vi "Main.vi"() -> ()   [LabVIEW 2015]
uses:
  TypeDefs/Queue Data.ctl
  FGV/Timer Actions.ctl
  SubVIs/App Data.vi
  SubVIs/App Strings.vi
panel:
  in  "Period [s]":dbl
  in  "Device name":tag="myDAQ1"
  out "Time Elapsed":dbl format="%<%M:%S>t"
  out "Status":string
  in  "Time [ms]":dbl
  in  "Frequency":dbl
  in  "Stop Button":bool
  in  "Acquire Button":bool
  out "Waveform Graph":dbl[](graph)
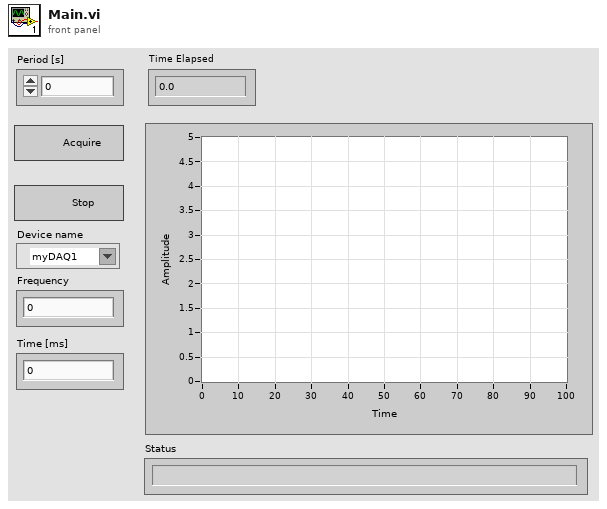
[diagram p1: front panel]
types:
  T1 = typedef "Timer Actions.ctl" = enum16{"Reset", "Get"}
  T2 = typedef "Queue Data.ctl" = cluster{"Action":string}
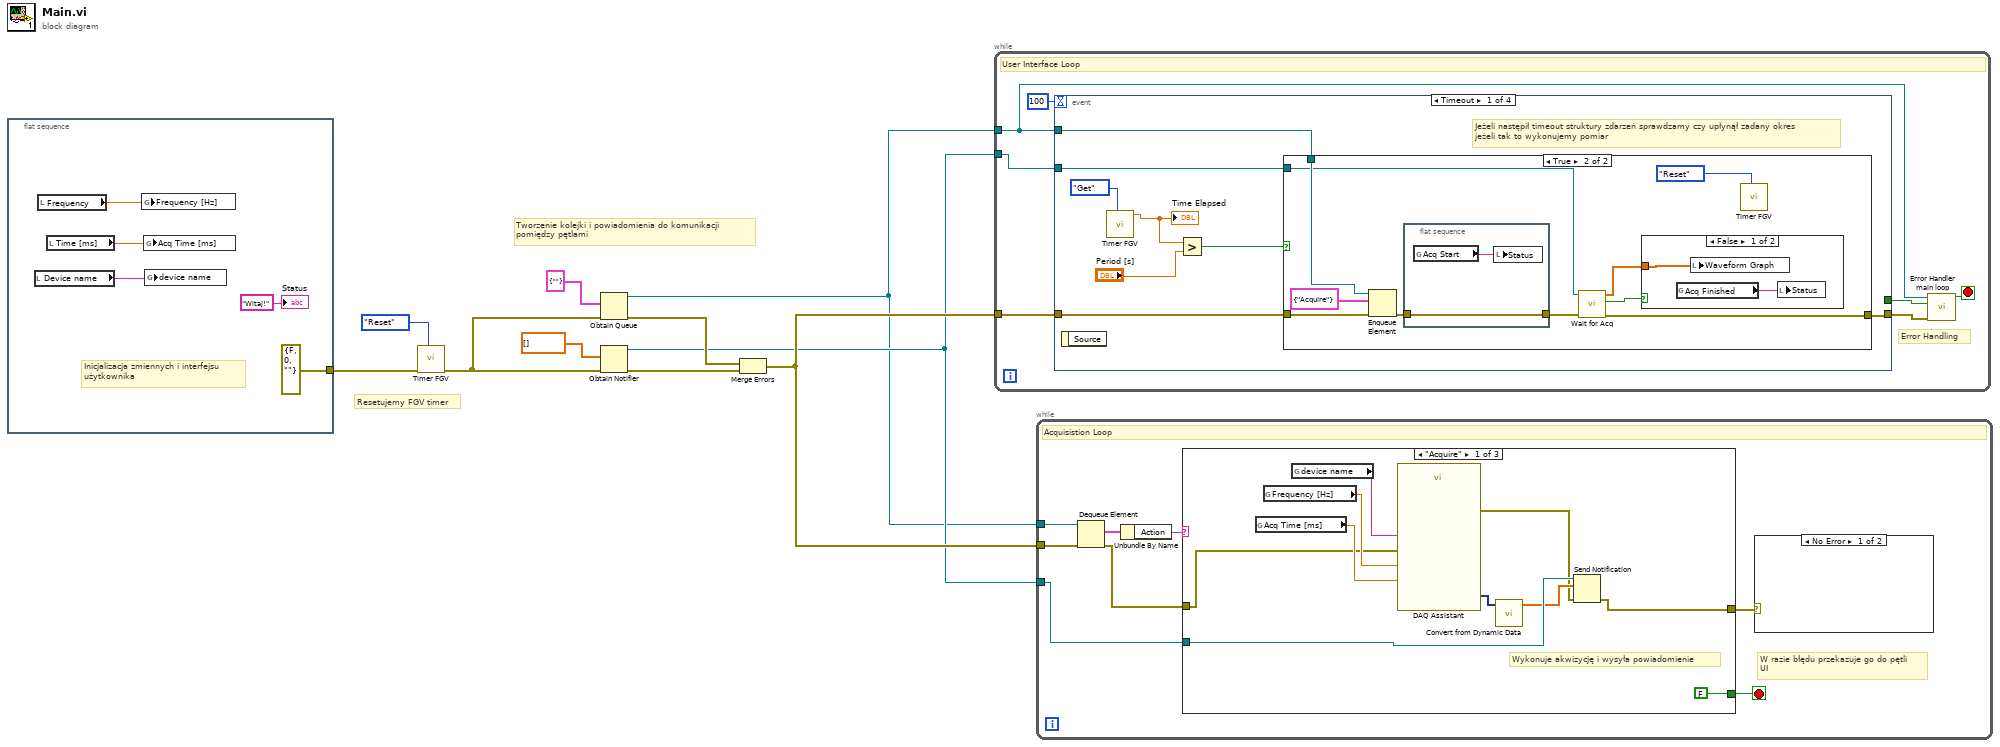
[diagram p0: block diagram]
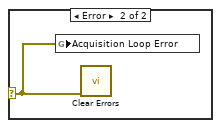
[diagram p2: hidden frame]
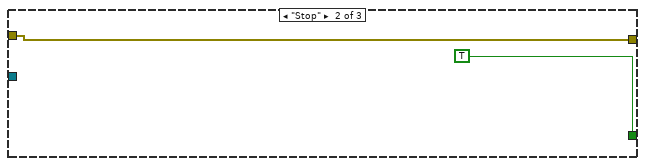
[diagram p3: hidden frame]
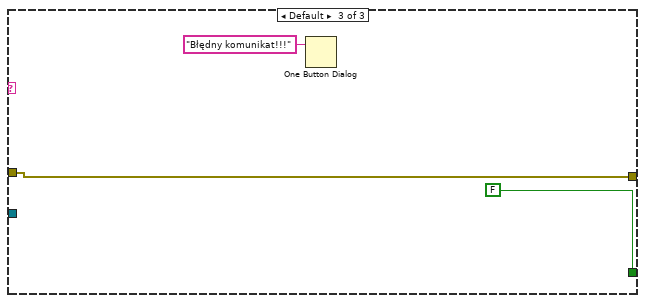
[diagram p4: hidden frame]
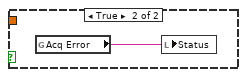
[diagram p6: hidden frame]
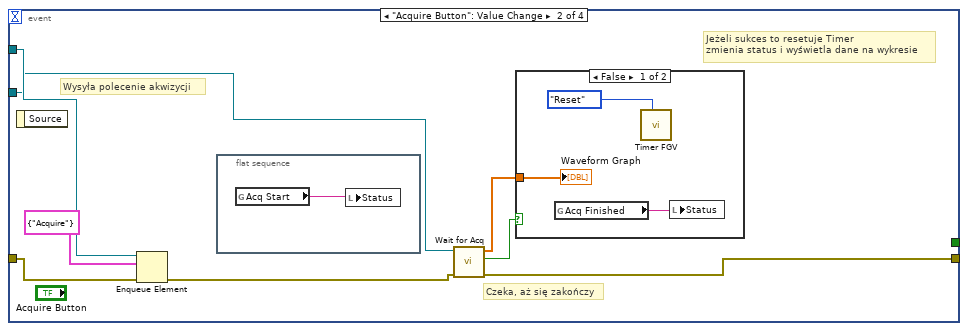
[diagram p7: hidden frame]
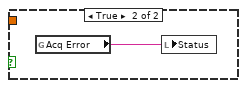
[diagram p8: hidden frame]
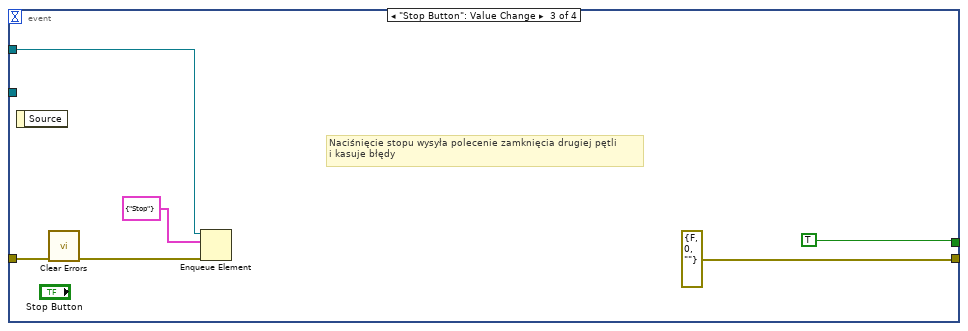
[diagram p9: hidden frame]
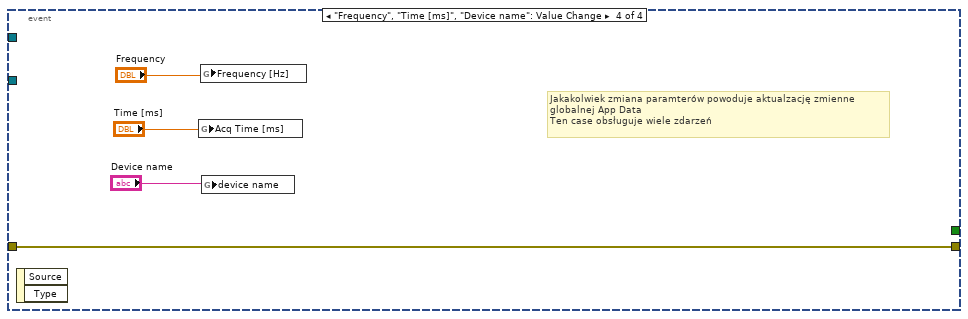
[diagram p10: hidden frame]
diagram:
  # "Resetujemy FGV timer"
  # "Tworzenie kolejki i powiadomienia do komunikacji \npomiędzy pętlami"
  n1 = flat-sequence {
    tunnel: [errorcluster {"status"=FALSE, "code"=0, "source"=""} ("error constant")] -> w3
    frame #0 {
      # "Inicjalizacja zmiennych i interfejsu \nużytkownika"
      n2 = local read "Device name"() -> (w11:tag)
      n3 = local read "Frequency"() -> (w13:dbl)
      n4 = local read "Time [ms]"() -> (w12:dbl)
      n5 = global write "App Data.vi" "Frequency [Hz]"(w13) -> ()
      n6 = global write "App Data.vi" "Acq Time [ms]"(w12) -> ()
      n7 = global write "App Data.vi" "device name"(w11) -> ()
      "Status" <- "Witaj!" ("Status")
    }
  }
  n8 = call "Timer FGV.vi"("Action"=Timer_Actions."Reset", "error in (no error)"=w3) -> ("error out"=w2:errorcluster)  [unwired: 8 in, 1 out]
  n9 = Obtain Queue(element data type=T2 {"Action"=""}, error in (no error)=w2) -> (queue out=w4:refnum<queue>, error out=w9:errorcluster)  [unwired: 3 in, 1 out]
  n10 = Obtain Notifier(notification data type=dbl[] [], error in (no error)=w2) -> (notifier out=w5:refnum<notifier>, error out=w7:errorcluster)  [unwired: 2 in, 1 out]
  n11 = Merge Errors(w9, w7) -> (w6:errorcluster)
  n12 = while {
    tunnel: w6 -> [w21]
    tunnel: w4 -> [w17]
    tunnel: w5 -> [w16]
    stop <- w18 stop-if-true
    # "Error Handling"
    # "User Interface Loop"
    n13 = event shown="[0] Timeout" {
      selector: _ -> [_ _ _ _]
      dyn-events: _ -> [_ _ _ _]
      timeout: 100 -> [_ _ _ _]
      tunnel: w21 -> [w28 w53 w62 w69]
      tunnel: [w27 w48 errorcluster {"status"=FALSE, "code"=0, "source"=""} ("error constant") w69] -> w19
      tunnel: [_ _ TRUE _] -> w20
      tunnel: w17 -> [w24 w54 w60 _]
      tunnel: w16 -> [w23 w50 _ _]
      event Timeout {
        # "Jeżeli następił timeout struktury zdarzeń sprawdzamy czy upłynął zadany okres \njeżeli tak to wykonujemy pomiar"
        n14 = event-data() -> ()  [unwired: 1 in, 1 out]
        n15 = call "Timer FGV.vi"("Action"=Timer_Actions."Get") -> ("Elapsed Time"=w26:dbl)  [unwired: 9 in, 1 out]
        "Time Elapsed" <- w26
        n16 = Greater?(x=w26, y="Period [s]") -> (0:w29:bool)
        n17 = case shown="True" w29 {
          tunnel: w28 -> [w31 w41]
          tunnel: [w31 w34] -> w27
          tunnel: w24 -> [_ w33]
          tunnel: w23 -> [_ w32]
          frame False {
          }
          frame True {
            n18 = Enqueue Element(queue=w33, element=T2 {"Action"="Acquire"}, error in (no error)=w41) -> (error out=w39:errorcluster)  [unwired: 1 in, 2 out]
            n19 = flat-sequence {
              tunnel: w39 -> [w45]
              tunnel: [w45] -> w38
              frame #0 {
                n20 = global read "App Strings.vi" "Acq Start"() -> (w46:string)
                n21 = local write "Status"(w46) -> ()
              }
            }
            n22 = call "Wait for Acq.vi"("error in (no error)"=w38, "Notifier in"=w32) -> ("error out"=w34:errorcluster, "timed out?"=w35:bool, "Array"=w37:dbl[])  [unwired: 7 in]
            n23 = case shown="False" w35 {
              tunnel: w37 -> [w42 _]
              frame False {
                n24 = global read "App Strings.vi" "Acq Finished"() -> (w43:string)
                n25 = local write "Waveform Graph"(w42) -> ()
                n26 = local write "Status"(w43) -> ()
              }
              frame True {
                n27 = global read "App Strings.vi" "Acq Error"() -> (w44:string)
                n28 = local write "Status"(w44) -> ()
              }
            }
            n29 = call "Timer FGV.vi"("Action"=Timer_Actions."Reset") -> ()  [unwired: 9 in, 2 out]
          }
        }
      }
      event "Acquire Button": Value Change {
        # "Jeżeli sukces to resetuje Timer\nzmienia status i wyświetla dane na wykresie"
        # "Czeka, aż się zakończy"
        # "Wysyła polecenie akwizycji"
        n30 = event-data() -> ()  [unwired: 1 in, 1 out]
        n31 = Enqueue Element(queue=w54, element=T2 {"Action"="Acquire"}, error in (no error)=w53) -> (error out=w49:errorcluster)  [unwired: 1 in, 2 out]
        n32 = flat-sequence {
          frame #0 {
            n33 = global read "App Strings.vi" "Acq Start"() -> (w55:string)
            n34 = local write "Status"(w55) -> ()
          }
        }
        n35 = call "Wait for Acq.vi"("error in (no error)"=w49, "Notifier in"=w50) -> ("error out"=w48:errorcluster, "timed out?"=w47:bool, "Array"=w51:dbl[])  [unwired: 7 in]
        n36 = case shown="False" w47 {
          tunnel: w51 -> [w56 _]
          frame False {
            n37 = global read "App Strings.vi" "Acq Finished"() -> (w58:string)
            n38 = call "Timer FGV.vi"("Action"=Timer_Actions."Reset") -> ()  [unwired: 9 in, 2 out]
            n39 = local write "Status"(w58) -> ()
            "Waveform Graph" <- w56
          }
          frame True {
            n40 = global read "App Strings.vi" "Acq Error"() -> (w59:string)
            n41 = local write "Status"(w59) -> ()
          }
        }
      }
      event "Stop Button": Value Change {
        # "Naciśnięcie stopu wysyła polecenie zamknięcia drugiej pętli\ni kasuje błędy"
        n42 = event-data() -> ()  [unwired: 1 in, 1 out]
        n43 = call <vilib>:"Clear Errors.vi"("error in (no error)"=w62) -> ("error out"=w61:errorcluster)  [unwired: 5 in, 1 out]
        n44 = Enqueue Element(queue=w60, element=T2 {"Action"="Stop"}, error in (no error)=w61) -> ()  [unwired: 1 in, 3 out]
      }
      event "Frequency", "Time [ms]", "Device name": Value Change {
        # "Jakakolwiek zmiana paramterów powoduje aktualzację zmienne \nglobalnej App Data\nTen case obsługuje wiele zdarzeń"
        n45 = event-data() -> ()  [unwired: 1 in, 2 out]
        n46 = global write "App Data.vi" "Acq Time [ms]"("Time [ms]") -> ()
        n47 = global write "App Data.vi" "Frequency [Hz]"("Frequency") -> ()
        n48 = global write "App Data.vi" "device name"("Device name") -> ()
      }
    }
    n49 = call "Error Handler main loop.vi"("error in (no error)"=w19, "Exit?"=w20, "Queue in"=w17) -> ("Exit?"=w18:bool)  [unwired: 8 in]
  }
  n50 = while {
    tunnel: w6 -> [w75]
    tunnel: w4 -> [w74]
    tunnel: w5 -> [w70]
    stop <- w72 stop-if-true
    # "W razie błędu przekazuje go do pętli\nUI"
    # "Acquisistion Loop"
    n51 = Dequeue Element(queue=w74, error in (no error)=w75) -> (element=w77:T2, error out=w73:errorcluster)  [unwired: 1 in, 2 out]
    n52 = Unbundle By Name(w77) -> ("Action"=w76:string)
    n53 = case shown="\"Acquire\"" w76 {
      tunnel: w73 -> [w84 w89 w92]
      tunnel: [FALSE TRUE FALSE] -> w72
      tunnel: [w79 w89 w92] -> w71
      tunnel: w70 -> [w82 _ _]
      frame "Acquire" {
        # "Wykonuje akwizycję i wysyła powiadomienie"
        n54 = global read "App Data.vi" "Acq Time [ms]"() -> (w85:dbl)
        n55 = global read "App Data.vi" "Frequency [Hz]"() -> (w86:dbl)
        n56 = global read "App Data.vi" "device name"() -> (w87:tag)
        n57 = call "DAQ Assistant"("rate"=w86, "timeout (s)"=w85, "error in"=w84, "device name"=w87) -> ("data"=w83:dynamicdata, "error out"=w80:errorcluster)  [unwired: 13 in, 1 out]
        n58 = call "Convert from Dynamic Data"("Dynamic Data Type"=w83) -> ("Array"=w81:dbl[])  [unwired: 3 in]
        n59 = Send Notification(notification=w81, notifier=w82, error in (no error)=w80) -> (error out=w79:errorcluster)  [unwired: 1 out]
      }
      frame "Stop" {
      }
      frame Default {
        n60 = One Button Dialog(message="Błędny komunikat!!!") -> ()  [unwired: 1 in, 1 out]
      }
    }
    n61 = case shown="No Error" w71 {
      selector: w71 -> [_ w78]
      frame No Error {
      }
      frame Error {
        n62 = global write "App Data.vi" "Acquisition Loop Error"(w78) -> ()
        n63 = call <vilib>:"Clear Errors.vi"("error in (no error)"=w78) -> ()  [unwired: 5 in, 2 out]
      }
    }
  }
